vi "LEBITplc.PenningSetValue.vi"(0 "i ref in":refnum<vi>, 1 "Nickname in":string, 2 "i attribute in":T1, 3 "value":dbl, 4 "index in":i32, 5 "error in":errorcluster) -> (13 "In Range?":bool, 14 "i ref out":refnum<vi>, 15 "Nicknames out":string[](array[string]), 16 "Index out":i32[](array[numeric]), 17 "values":dbl[](array[numeric]), 18 "Log Out?":bool[](array[boolean]), 19 "error out":errorcluster)   [LabVIEW 2014, in "LEBITplc.lvlib"]
uses:
  LEBITplc.lvlib
  LEBITplc.i attribute.ctl
panel:
  in  "file path":path=path "\\\\Projects\\proj1/lebit/Data Exchange/data/IonGuideControl/Conversion/MassConversion.txt"
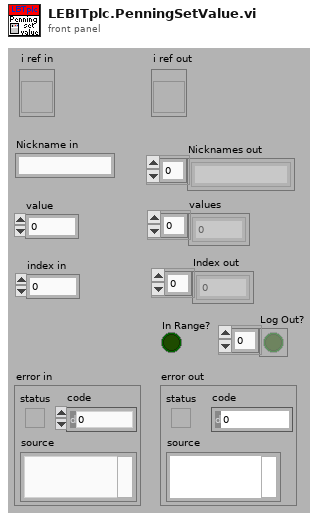
[diagram p1: front panel]
types:
  T1 = typedef "LEBITplc.lvlib/LEBITplc.i attribute.ctl" = cluster{"LLFLocation":string, "SetFileLocation":string, "nickNames":string[], "setValuePLCServiceID":i32[], "GUIServiceID":i32[], "monValuePLC":string[], "SetValueServiceID":i32[], "MonValueServiceID":i32[], "SetValue":dbl[][], "SetValueMin":dbl[], "SetValueMax":dbl[], "SetValueInfoServiceID":i32[], "GUINames":string[], "ListOfBases":string[], "Scale":dbl[], "Offset":dbl[], "setValuePLC":string[], "BaseName":string[], "ScaleServiceID":i32[], "OffsetServiceID":i32[], "AllPLCValues":string[], "CondSpecialArray":string[][], "CondSpecialIndex":i32[], "CondSpecialMonValue":dbl[], "RecentlyChanged":i32[], "SetFileLocationID":i32, "Dependent-Monitors":string[][], "LastLoadedFiles":string[], "IonGuideCalibLocation":string, "Monitor Dependent":string[], "Special":string[], "PLC?":bool[], "Start Date":string, "ListOfBasesServiceID":i32, "SETRA VISA resource":refnum<visa-resource-name>}
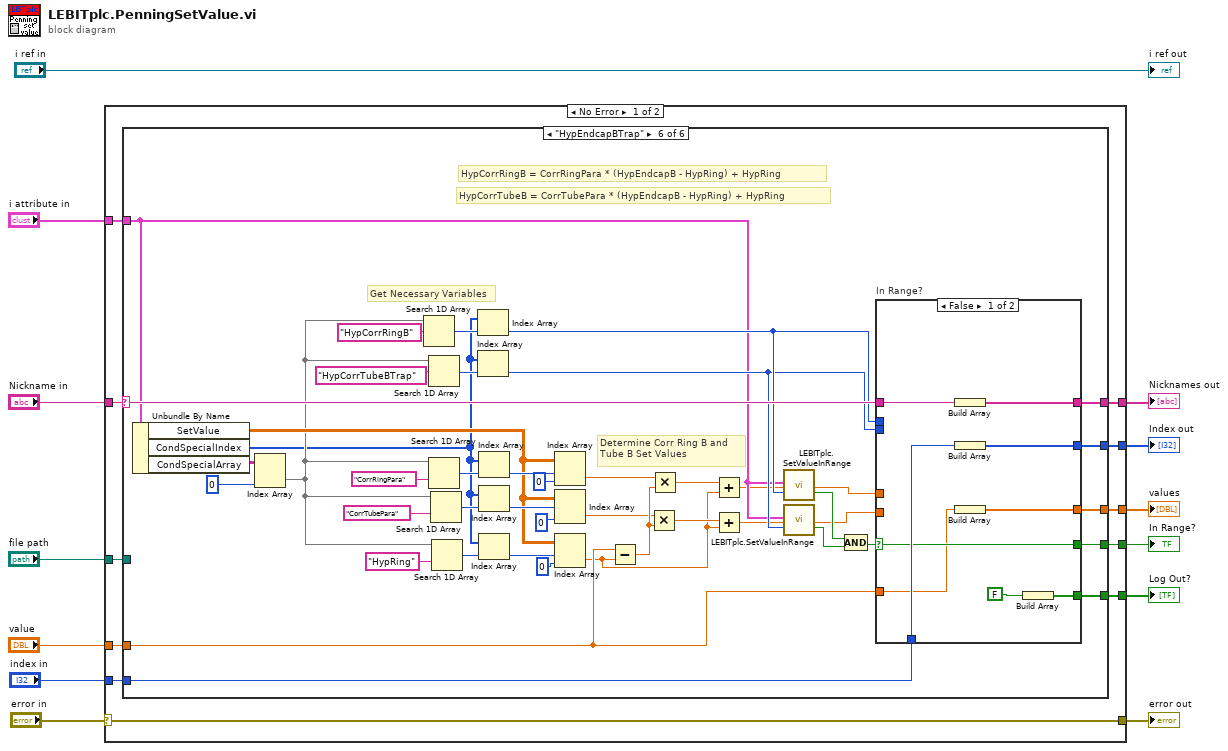
[diagram p0: block diagram]
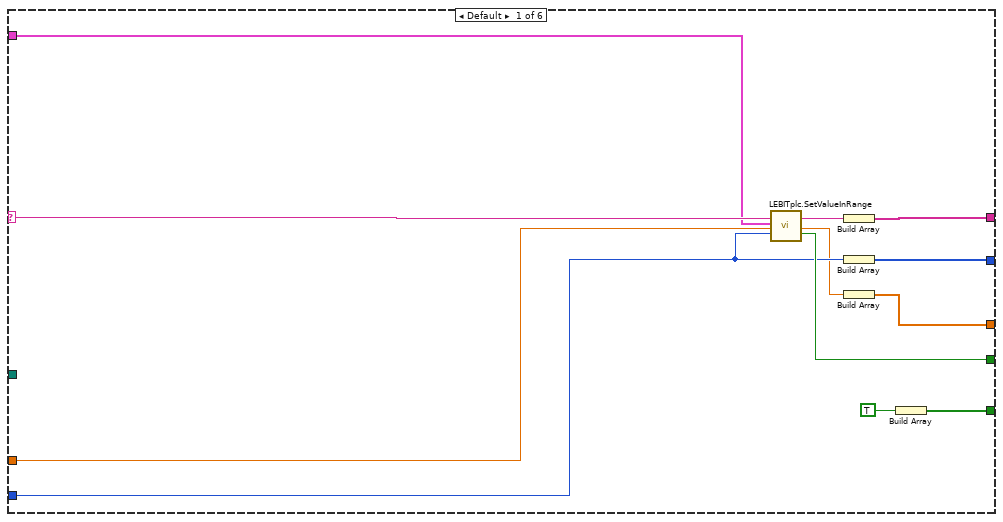
[diagram p2: hidden frame]
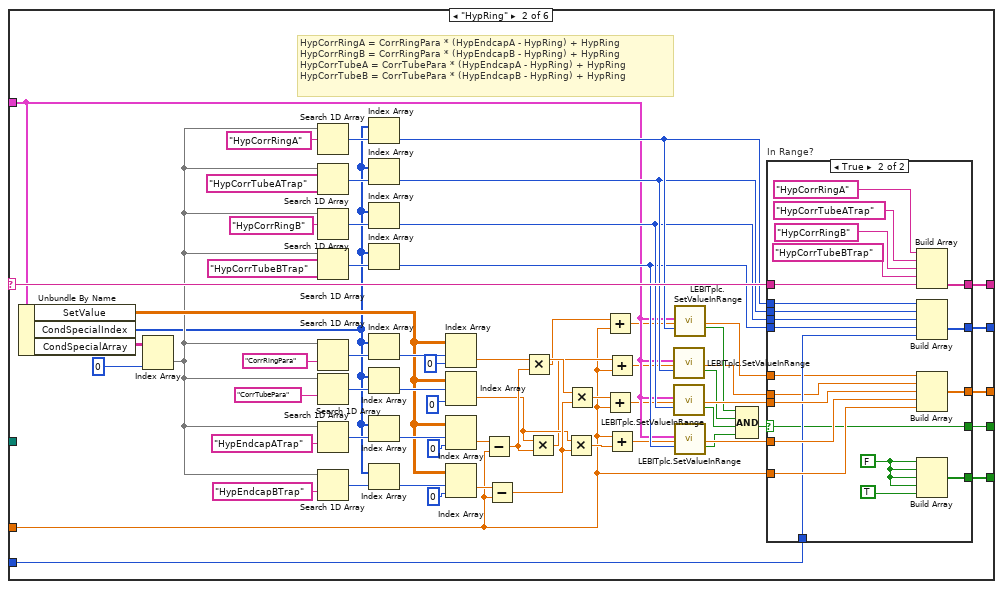
[diagram p3: hidden frame]
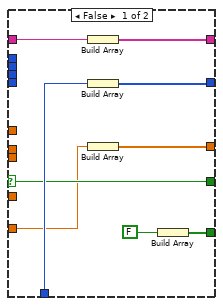
[diagram p4: hidden frame]
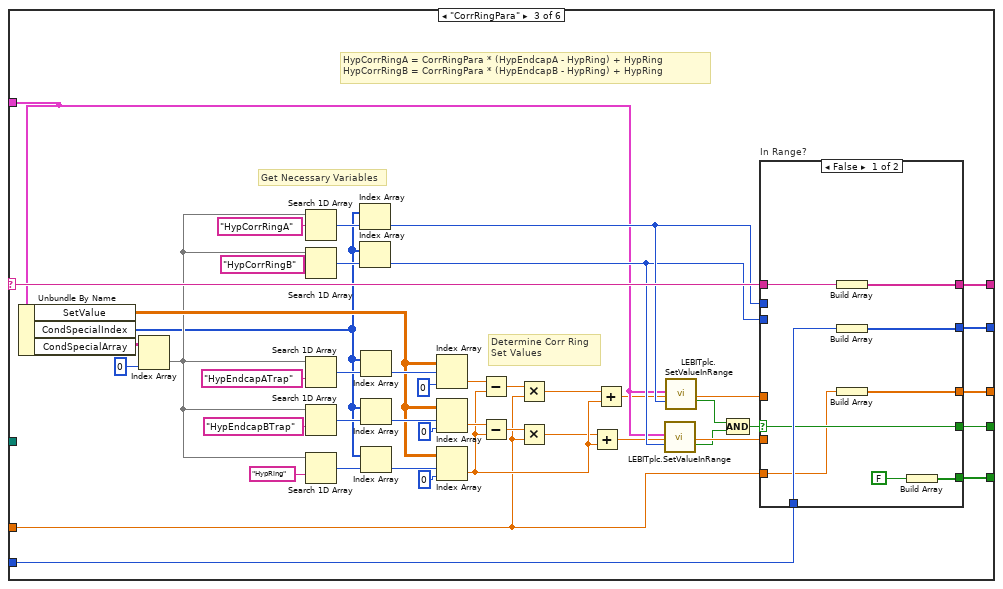
[diagram p5: hidden frame]
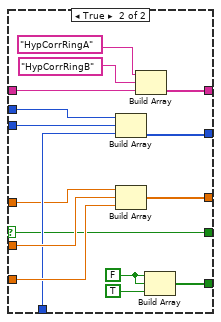
[diagram p6: hidden frame]
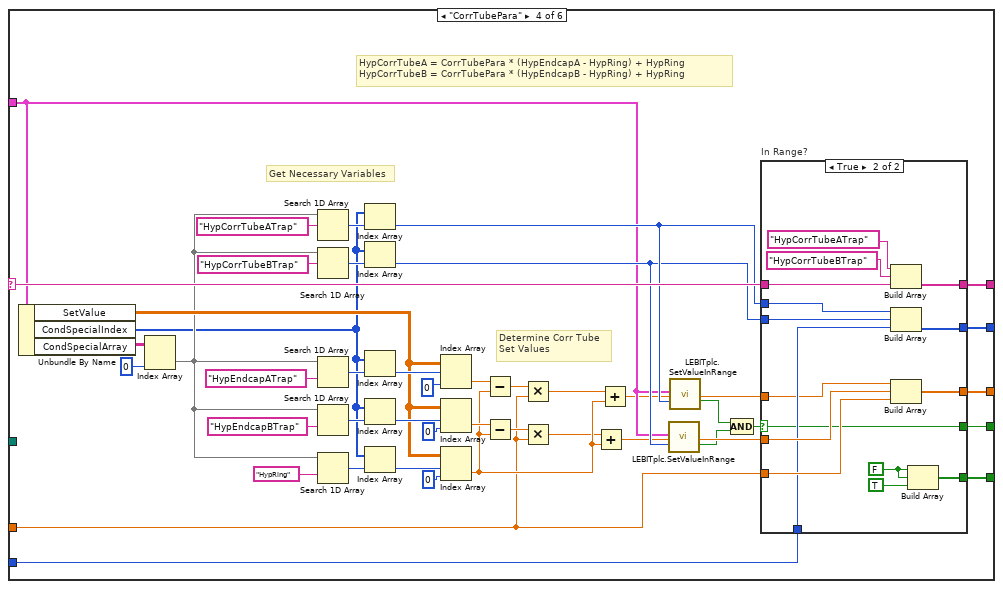
[diagram p7: hidden frame]
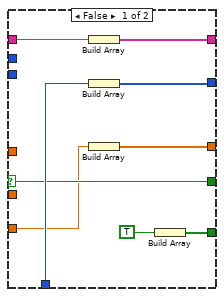
[diagram p8: hidden frame]
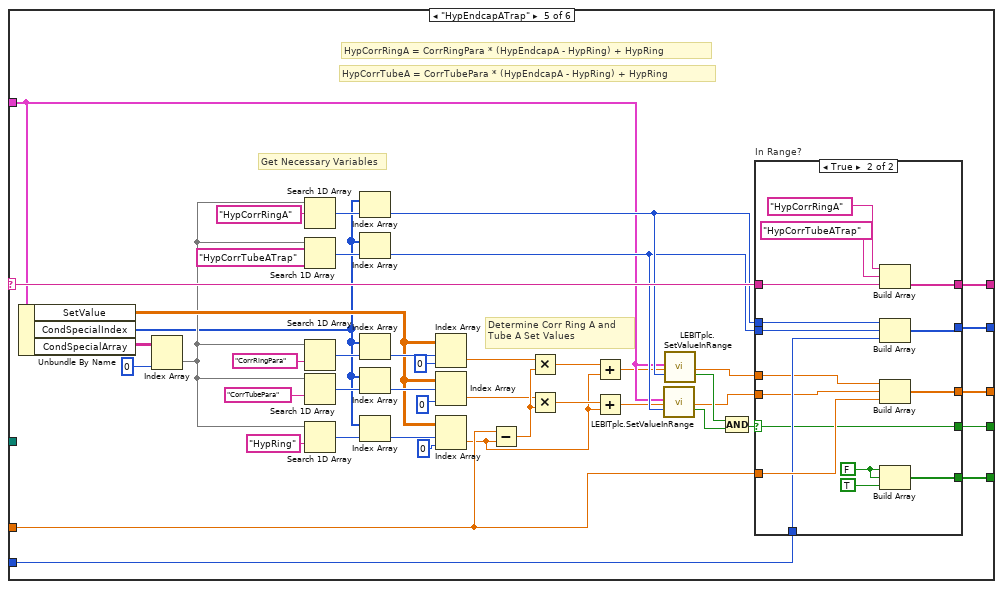
[diagram p9: hidden frame]
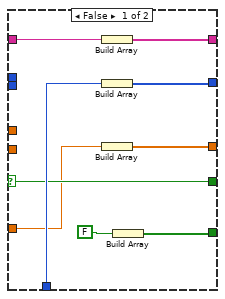
[diagram p10: hidden frame]
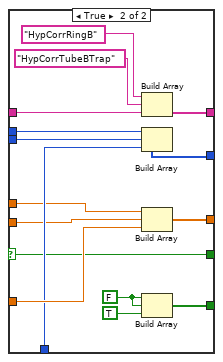
[diagram p11: hidden frame]
diagram:
  n1 = case shown="No Error" "error in" {
    selector: "error in" -> [w15 w415]
    tunnel: "Nickname in" -> [w24 _]
    tunnel: "i attribute in" -> [w23 _]
    tunnel: "value" -> [w22 _]
    tunnel: [w21 _] -> w10
    tunnel: [w20 _] -> w9
    tunnel: "file path" -> [w19 _]
    tunnel: "index in" -> [w18 _]
    tunnel: [w17 _] -> w6
    tunnel: [w16 _] -> w5
    tunnel: [w15 w415] -> w3
    tunnel: [w14 _] -> w1
    frame No Error {
      n2 = case shown="\"HypEndcapBTrap\"" w24 {
        selector: w24 -> [w32 w92 w172 w243 w312 w382]
        tunnel: w23 -> [w27 w50 w149 w220 w285 w355]
        tunnel: w22 -> [w30 w45 w134 w205 w277 w347]
        tunnel: [w36 w93 w173 w244 w313 w383] -> w21
        tunnel: [w35 w91 w171 w242 w311 w381] -> w20
        tunnel: w19 -> [_ _ _ _ _ _]
        tunnel: w18 -> [w31 w78 w162 w233 w302 w372]
        tunnel: [w34 w79 w163 w234 w303 w373] -> w17
        tunnel: [w33 w76 w160 w231 w300 w370] -> w16
        tunnel: [w25 w37 w133 w204 w275 w345] -> w14
        frame Default {
          n3 = call "LEBITplc.SetValueInRange.vi"("CommandName in"=w32, "i attribute in"=w27, "value in"=w30, "index of element"=w31) -> ("CommandName out"=w28:string, "value out"=w29:dbl, "In Range?"=w33:bool)  [unwired: 11 in, 2 out]
          n4 = Build Array(w28) -> (w35:string[])
          n5 = Build Array(w31) -> (w34:i32[])
          n6 = Build Array(w29) -> (w36:dbl[])
          n7 = Build Array(TRUE) -> (w25:bool[])
        }
        frame "HypRing" {
          # "HypCorrRingA = CorrRingPara * (HypEndcapA - HypRing) + HypRing\nHypCorrRingB = CorrRingPara * (HypEndcapB - HypRing) + HypRing\nHypCorrTubeA = CorrTubePara * (HypEndcapA - HypRing) + HypRing\nHypCorrTubeB = CorrTubePara * (HypEndcapB - HypRing) + HypRing"
          n8 = Unbundle By Name(w50) -> ("SetValue"=w71:dbl[][], "CondSpecialIndex"=w65:i32[], "CondSpecialArray"=w90:string[][])
          n9 = Index Array(array=w90, index (col)=0 ("index (row)")) -> (element=w66:string[])  [unwired: 1 in]
          n10 = Search 1D Array(1D array=w66, element="HypCorrRingA") -> (index of element=w68:i32)  [unwired: 1 in]
          n11 = Search 1D Array(1D array=w66, element="HypCorrTubeATrap") -> (index of element=w70:i32)  [unwired: 1 in]
          n12 = Search 1D Array(1D array=w66, element="HypCorrRingB") -> (index of element=w81:i32)  [unwired: 1 in]
          n13 = Search 1D Array(1D array=w66, element="HypCorrTubeBTrap") -> (index of element=w83:i32)  [unwired: 1 in]
          n14 = Search 1D Array(1D array=w66, element="CorrRingPara") -> (index of element=w89:i32)  [unwired: 1 in]
          n15 = Search 1D Array(1D array=w66, element="CorrTubePara") -> (index of element=w88:i32)  [unwired: 1 in]
          n16 = Search 1D Array(1D array=w66, element="HypEndcapATrap") -> (index of element=w87:i32)  [unwired: 1 in]
          n17 = Search 1D Array(1D array=w66, element="HypEndcapBTrap") -> (index of element=w73:i32)  [unwired: 1 in]
          n18 = Index Array(array=w65, index=w68) -> (element=w54:i32)
          n19 = Index Array(array=w65, index=w70) -> (element=w53:i32)
          n20 = Index Array(array=w65, index=w81) -> (element=w52:i32)
          n21 = Index Array(array=w65, index=w83) -> (element=w51:i32)
          n22 = Index Array(array=w65, index=w89) -> (element=w84:i32)
          n23 = Index Array(array=w65, index=w88) -> (element=w85:i32)
          n24 = Index Array(array=w65, index=w87) -> (element=w86:i32)
          n25 = Index Array(array=w65, index=w73) -> (element=w72:i32)
          n26 = Index Array(array=w71, index (row)=w84, index (col)=0 ("disabled index (col)")) -> (element=w62:dbl)
          n27 = Index Array(array=w71, index (row)=w85, index (col)=0 ("disabled index (col)")) -> (element=w59:dbl)
          n28 = Index Array(array=w71, index (row)=w86, index (col)=0 ("disabled index (col)")) -> (element=w63:dbl)
          n29 = Index Array(array=w71, index (row)=w72, index (col)=0 ("disabled index (col)")) -> (element=w64:dbl)
          n30 = Subtract(x=w63, y=w45) -> (x-y=w61:dbl)
          n31 = Subtract(x=w64, y=w45) -> (x-y=w60:dbl)
          n32 = Multiply(x=w62, y=w61) -> (x*y=w56:dbl)
          n33 = Multiply(x=w59, y=w61) -> (x*y=w55:dbl)
          n34 = Multiply(x=w59, y=w60) -> (x*y=w57:dbl)
          n35 = Multiply(x=w62, y=w60) -> (x*y=w58:dbl)
          n36 = Add(x=w56, y=w45) -> (x+y=w49:dbl)
          n37 = Add(x=w58, y=w45) -> (x+y=w47:dbl)
          n38 = Add(x=w55, y=w45) -> (x+y=w48:dbl)
          n39 = Add(x=w45, y=w57) -> (x+y=w46:dbl)
          n40 = call "LEBITplc.SetValueInRange.vi"("i attribute in"=w50, "value in"=w48, "index of element"=w53) -> ("value out"=w38:dbl, "In Range?"=w42:bool)  [unwired: 12 in, 3 out]
          n41 = call "LEBITplc.SetValueInRange.vi"("i attribute in"=w50, "value in"=w47, "index of element"=w52) -> ("value out"=w94:dbl, "In Range?"=w41:bool)  [unwired: 12 in, 3 out]
          n42 = call "LEBITplc.SetValueInRange.vi"("i attribute in"=w50, "value in"=w49, "index of element"=w54) -> ("value out"=w39:dbl, "In Range?"=w43:bool)  [unwired: 12 in, 3 out]
          n43 = call "LEBITplc.SetValueInRange.vi"("i attribute in"=w50, "value in"=w46, "index of element"=w51) -> ("value out"=w95:dbl, "In Range?"=w40:bool)  [unwired: 12 in, 3 out]
          n44 = Compound Arithmetic op=AND(w43, w42, w41, w40) -> (w44:bool)
          n45 = case "In Range?" shown="True" w44 {
            selector: w44 -> [w106 w124]
            tunnel: w45 -> [w105 w130]
            tunnel: w95 -> [_ w131]
            tunnel: w94 -> [_ w132]
            tunnel: [w104 w129] -> w93
            tunnel: w92 -> [w109 w128]
            tunnel: [w110 w127] -> w91
            tunnel: [w108 w126] -> w79
            tunnel: w78 -> [w107 w125]
            tunnel: [w106 w124] -> w76
            tunnel: w54 -> [_ w119]
            tunnel: w53 -> [_ w118]
            tunnel: w52 -> [_ w117]
            tunnel: w51 -> [_ w116]
            tunnel: w39 -> [_ w115]
            tunnel: w38 -> [_ w114]
            tunnel: [w102 w111] -> w37
            frame False {
              n46 = Build Array(w109) -> (w110:string[])
              n47 = Build Array(w107) -> (w108:i32[])
              n48 = Build Array(w105) -> (w104:dbl[])
              n49 = Build Array(FALSE) -> (w102:bool[])
            }
            frame True {
              w112 = FALSE
              n50 = Build Array("HypCorrRingA" ("element"), "HypCorrTubeATrap" ("element"), "HypCorrRingB" ("element"), "HypCorrTubeBTrap" ("element"), w128) -> (w127:string[])
              n51 = Build Array(w119, w118, w117, w116, w125) -> (w126:i32[])
              n52 = Build Array(w115, w114, w132, w131, w130) -> (w129:dbl[])
              n53 = Build Array(w112, w112, w112, w112, TRUE) -> (w111:bool[])
            }
          }
        }
        frame "CorrRingPara" {
          # "HypCorrRingA = CorrRingPara * (HypEndcapA - HypRing) + HypRing\nHypCorrRingB = CorrRingPara * (HypEndcapB - HypRing) + HypRing"
          # "Determine Corr Ring\nSet Values"
          # "Get Necessary Variables"
          n54 = Unbundle By Name(w149) -> ("SetValue"=w155:dbl[][], "CondSpecialIndex"=w142:i32[], "CondSpecialArray"=w170:string[][])
          n55 = Index Array(array=w170, index (col)=0 ("index (row)")) -> (element=w152:string[])  [unwired: 1 in]
          n56 = Search 1D Array(1D array=w152, element="HypCorrRingA") -> (index of element=w154:i32)  [unwired: 1 in]
          n57 = Search 1D Array(1D array=w152, element="HypCorrRingB") -> (index of element=w165:i32)  [unwired: 1 in]
          n58 = Search 1D Array(1D array=w152, element="HypEndcapATrap") -> (index of element=w169:i32)  [unwired: 1 in]
          n59 = Search 1D Array(1D array=w152, element="HypEndcapBTrap") -> (index of element=w168:i32)  [unwired: 1 in]
          n60 = Search 1D Array(1D array=w152, element="HypRing") -> (index of element=w157:i32)  [unwired: 1 in]
          n61 = Index Array(array=w142, index=w154) -> (element=w151:i32)
          n62 = Index Array(array=w142, index=w165) -> (element=w150:i32)
          n63 = Index Array(array=w142, index=w169) -> (element=w166:i32)
          n64 = Index Array(array=w142, index=w168) -> (element=w167:i32)
          n65 = Index Array(array=w142, index=w157) -> (element=w156:i32)
          n66 = Index Array(array=w155, index (row)=w166, index (col)=0 ("disabled index (col)")) -> (element=w141:dbl)
          n67 = Index Array(array=w155, index (row)=w167, index (col)=0 ("disabled index (col)")) -> (element=w140:dbl)
          n68 = Index Array(array=w155, index (row)=w156, index (col)=0 ("disabled index (col)")) -> (element=w139:dbl)
          n69 = Subtract(x=w141, y=w139) -> (x-y=w138:dbl)
          n70 = Subtract(x=w140, y=w139) -> (x-y=w137:dbl)
          n71 = Multiply(x=w138, y=w134) -> (x*y=w136:dbl)
          n72 = Multiply(x=w137, y=w134) -> (x*y=w135:dbl)
          n73 = Add(x=w135, y=w139) -> (x+y=w147:dbl)
          n74 = Add(x=w136, y=w139) -> (x+y=w148:dbl)
          n75 = call "LEBITplc.SetValueInRange.vi"("i attribute in"=w149, "value in"=w147, "index of element"=w150) -> ("value out"=w174:dbl, "In Range?"=w144:bool)  [unwired: 12 in, 3 out]
          n76 = call "LEBITplc.SetValueInRange.vi"("i attribute in"=w149, "value in"=w148, "index of element"=w151) -> ("value out"=w143:dbl, "In Range?"=w145:bool)  [unwired: 12 in, 3 out]
          n77 = Compound Arithmetic op=AND(w145, w144) -> (w146:bool)
          n78 = case "In Range?" shown="False" w146 {
            selector: w146 -> [w183 w196]
            tunnel: w134 -> [w182 w202]
            tunnel: w174 -> [_ w203]
            tunnel: [w181 w201] -> w173
            tunnel: w172 -> [w186 w200]
            tunnel: [w187 w199] -> w171
            tunnel: [w185 w198] -> w163
            tunnel: w162 -> [w184 w197]
            tunnel: [w183 w196] -> w160
            tunnel: w151 -> [_ w193]
            tunnel: w150 -> [_ w192]
            tunnel: w143 -> [_ w191]
            tunnel: [w179 w188] -> w133
            frame False {
              n79 = Build Array(w186) -> (w187:string[])
              n80 = Build Array(w184) -> (w185:i32[])
              n81 = Build Array(w182) -> (w181:dbl[])
              n82 = Build Array(FALSE) -> (w179:bool[])
            }
            frame True {
              w189 = FALSE
              n83 = Build Array(w193, w192, w197) -> (w198:i32[])
              n84 = Build Array(w191, w203, w202) -> (w201:dbl[])
              n85 = Build Array("HypCorrRingA" ("element"), "HypCorrRingB" ("element"), w200) -> (w199:string[])
              n86 = Build Array(w189, w189, TRUE) -> (w188:bool[])
            }
          }
        }
        frame "CorrTubePara" {
          # "HypCorrTubeA = CorrTubePara * (HypEndcapA - HypRing) + HypRing\nHypCorrTubeB = CorrTubePara * (HypEndcapB - HypRing) + HypRing"
          # "Determine Corr Tube\nSet Values"
          # "Get Necessary Variables"
          n87 = Unbundle By Name(w220) -> ("SetValue"=w226:dbl[][], "CondSpecialIndex"=w213:i32[], "CondSpecialArray"=w241:string[][])
          n88 = Index Array(array=w241, index (col)=0 ("index (row)")) -> (element=w223:string[])  [unwired: 1 in]
          n89 = Search 1D Array(1D array=w223, element="HypCorrTubeATrap") -> (index of element=w225:i32)  [unwired: 1 in]
          n90 = Search 1D Array(1D array=w223, element="HypCorrTubeBTrap") -> (index of element=w236:i32)  [unwired: 1 in]
          n91 = Search 1D Array(1D array=w223, element="HypEndcapATrap") -> (index of element=w240:i32)  [unwired: 1 in]
          n92 = Search 1D Array(1D array=w223, element="HypEndcapBTrap") -> (index of element=w239:i32)  [unwired: 1 in]
          n93 = Search 1D Array(1D array=w223, element="HypRing") -> (index of element=w228:i32)  [unwired: 1 in]
          n94 = Index Array(array=w213, index=w225) -> (element=w222:i32)
          n95 = Index Array(array=w213, index=w236) -> (element=w221:i32)
          n96 = Index Array(array=w213, index=w240) -> (element=w237:i32)
          n97 = Index Array(array=w213, index=w239) -> (element=w238:i32)
          n98 = Index Array(array=w213, index=w228) -> (element=w227:i32)
          n99 = Index Array(array=w226, index (row)=w237, index (col)=0 ("disabled index (col)")) -> (element=w212:dbl)
          n100 = Index Array(array=w226, index (row)=w238, index (col)=0 ("disabled index (col)")) -> (element=w211:dbl)
          n101 = Index Array(array=w226, index (row)=w227, index (col)=0 ("disabled index (col)")) -> (element=w210:dbl)
          n102 = Subtract(x=w212, y=w210) -> (x-y=w209:dbl)
          n103 = Subtract(x=w211, y=w210) -> (x-y=w208:dbl)
          n104 = Multiply(x=w209, y=w205) -> (x*y=w207:dbl)
          n105 = Multiply(x=w208, y=w205) -> (x*y=w206:dbl)
          n106 = Add(x=w206, y=w210) -> (x+y=w218:dbl)
          n107 = Add(x=w207, y=w210) -> (x+y=w219:dbl)
          n108 = call "LEBITplc.SetValueInRange.vi"("i attribute in"=w220, "value in"=w218, "index of element"=w221) -> ("value out"=w245:dbl, "In Range?"=w215:bool)  [unwired: 12 in, 3 out]
          n109 = call "LEBITplc.SetValueInRange.vi"("i attribute in"=w220, "value in"=w219, "index of element"=w222) -> ("value out"=w214:dbl, "In Range?"=w216:bool)  [unwired: 12 in, 3 out]
          n110 = Compound Arithmetic op=AND(w216, w215) -> (w217:bool)
          n111 = case "In Range?" shown="True" w217 {
            selector: w217 -> [w254 w267]
            tunnel: w205 -> [w253 w273]
            tunnel: w245 -> [_ w274]
            tunnel: [w252 w272] -> w244
            tunnel: w243 -> [w257 w271]
            tunnel: [w258 w270] -> w242
            tunnel: [w256 w269] -> w234
            tunnel: w233 -> [w255 w268]
            tunnel: [w254 w267] -> w231
            tunnel: w222 -> [_ w264]
            tunnel: w221 -> [_ w263]
            tunnel: w214 -> [_ w262]
            tunnel: [w250 w259] -> w204
            frame False {
              n112 = Build Array(w257) -> (w258:string[])
              n113 = Build Array(w255) -> (w256:i32[])
              n114 = Build Array(w253) -> (w252:dbl[])
              n115 = Build Array(TRUE) -> (w250:bool[])
            }
            frame True {
              w260 = FALSE
              n116 = Build Array("HypCorrTubeATrap" ("element"), "HypCorrTubeBTrap" ("element"), w271) -> (w270:string[])
              n117 = Build Array(w264, w263, w268) -> (w269:i32[])
              n118 = Build Array(w262, w274, w273) -> (w272:dbl[])
              n119 = Build Array(w260, w260, TRUE) -> (w259:bool[])
            }
          }
        }
        frame "HypEndcapATrap" {
          # "HypCorrTubeA = CorrTubePara * (HypEndcapA - HypRing) + HypRing"
          # "HypCorrRingA = CorrRingPara * (HypEndcapA - HypRing) + HypRing"
          # "Determine Corr Ring A and \nTube A Set Values"
          # "Get Necessary Variables"
          n120 = Unbundle By Name(w285) -> ("SetValue"=w299:dbl[][], "CondSpecialIndex"=w293:i32[], "CondSpecialArray"=w310:string[][])
          n121 = Index Array(array=w310, index (col)=0 ("index (row)")) -> (element=w294:string[])  [unwired: 1 in]
          n122 = Search 1D Array(1D array=w294, element="HypCorrRingA") -> (index of element=w296:i32)  [unwired: 1 in]
          n123 = Search 1D Array(1D array=w294, element="HypCorrTubeATrap") -> (index of element=w298:i32)  [unwired: 1 in]
          n124 = Search 1D Array(1D array=w294, element="CorrRingPara") -> (index of element=w309:i32)  [unwired: 1 in]
          n125 = Search 1D Array(1D array=w294, element="CorrTubePara") -> (index of element=w308:i32)  [unwired: 1 in]
          n126 = Search 1D Array(1D array=w294, element="HypRing") -> (index of element=w307:i32)  [unwired: 1 in]
          n127 = Index Array(array=w293, index=w296) -> (element=w287:i32)
          n128 = Index Array(array=w293, index=w298) -> (element=w286:i32)
          n129 = Index Array(array=w293, index=w309) -> (element=w304:i32)
          n130 = Index Array(array=w293, index=w308) -> (element=w305:i32)
          n131 = Index Array(array=w293, index=w307) -> (element=w306:i32)
          n132 = Index Array(array=w299, index (row)=w304, index (col)=0 ("disabled index (col)")) -> (element=w292:dbl)
          n133 = Index Array(array=w299, index (row)=w305, index (col)=0 ("disabled index (col)")) -> (element=w290:dbl)
          n134 = Index Array(array=w299, index (row)=w306, index (col)=0 ("disabled index (col)")) -> (element=w276:dbl)
          n135 = Subtract(x=w277, y=w276) -> (x-y=w291:dbl)
          n136 = Multiply(x=w292, y=w291) -> (x*y=w289:dbl)
          n137 = Multiply(x=w290, y=w291) -> (x*y=w288:dbl)
          n138 = Add(x=w289, y=w276) -> (x+y=w284:dbl)
          n139 = Add(x=w288, y=w276) -> (x+y=w283:dbl)
          n140 = call "LEBITplc.SetValueInRange.vi"("i attribute in"=w285, "value in"=w283, "index of element"=w286) -> ("value out"=w278:dbl, "In Range?"=w280:bool)  [unwired: 12 in, 3 out]
          n141 = call "LEBITplc.SetValueInRange.vi"("i attribute in"=w285, "value in"=w284, "index of element"=w287) -> ("value out"=w279:dbl, "In Range?"=w281:bool)  [unwired: 12 in, 3 out]
          n142 = Compound Arithmetic op=AND(w281, w280) -> (w282:bool)
          n143 = case "In Range?" shown="True" w282 {
            selector: w282 -> [w324 w338]
            tunnel: w277 -> [w323 w344]
            tunnel: [w322 w343] -> w313
            tunnel: w312 -> [w327 w342]
            tunnel: [w328 w341] -> w311
            tunnel: [w326 w340] -> w303
            tunnel: w302 -> [w325 w339]
            tunnel: [w324 w338] -> w300
            tunnel: w287 -> [_ w335]
            tunnel: w286 -> [_ w334]
            tunnel: w279 -> [_ w333]
            tunnel: w278 -> [_ w332]
            tunnel: [w321 w329] -> w275
            frame False {
              n144 = Build Array(w327) -> (w328:string[])
              n145 = Build Array(w325) -> (w326:i32[])
              n146 = Build Array(w323) -> (w322:dbl[])
              n147 = Build Array(FALSE) -> (w321:bool[])
            }
            frame True {
              w330 = FALSE
              n148 = Build Array("HypCorrRingA" ("element"), "HypCorrTubeATrap" ("element"), w342) -> (w341:string[])
              n149 = Build Array(w335, w334, w339) -> (w340:i32[])
              n150 = Build Array(w333, w332, w344) -> (w343:dbl[])
              n151 = Build Array(w330, w330, TRUE) -> (w329:bool[])
            }
          }
        }
        frame "HypEndcapBTrap" {
          # "HypCorrTubeB = CorrTubePara * (HypEndcapB - HypRing) + HypRing"
          # "HypCorrRingB = CorrRingPara * (HypEndcapB - HypRing) + HypRing"
          # "Determine Corr Ring B and \nTube B Set Values"
          # "Get Necessary Variables"
          n152 = Unbundle By Name(w355) -> ("SetValue"=w369:dbl[][], "CondSpecialIndex"=w363:i32[], "CondSpecialArray"=w380:string[][])
          n153 = Index Array(array=w380, index (col)=0 ("index (row)")) -> (element=w364:string[])  [unwired: 1 in]
          n154 = Search 1D Array(1D array=w364, element="HypCorrRingB") -> (index of element=w366:i32)  [unwired: 1 in]
          n155 = Search 1D Array(1D array=w364, element="HypCorrTubeBTrap") -> (index of element=w368:i32)  [unwired: 1 in]
          n156 = Search 1D Array(1D array=w364, element="CorrRingPara") -> (index of element=w379:i32)  [unwired: 1 in]
          n157 = Search 1D Array(1D array=w364, element="CorrTubePara") -> (index of element=w378:i32)  [unwired: 1 in]
          n158 = Search 1D Array(1D array=w364, element="HypRing") -> (index of element=w377:i32)  [unwired: 1 in]
          n159 = Index Array(array=w363, index=w366) -> (element=w357:i32)
          n160 = Index Array(array=w363, index=w368) -> (element=w356:i32)
          n161 = Index Array(array=w363, index=w379) -> (element=w374:i32)
          n162 = Index Array(array=w363, index=w378) -> (element=w375:i32)
          n163 = Index Array(array=w363, index=w377) -> (element=w376:i32)
          n164 = Index Array(array=w369, index (row)=w374, index (col)=0 ("disabled index (col)")) -> (element=w362:dbl)
          n165 = Index Array(array=w369, index (row)=w375, index (col)=0 ("disabled index (col)")) -> (element=w360:dbl)
          n166 = Index Array(array=w369, index (row)=w376, index (col)=0 ("disabled index (col)")) -> (element=w346:dbl)
          n167 = Subtract(x=w347, y=w346) -> (x-y=w361:dbl)
          n168 = Multiply(x=w360, y=w361) -> (x*y=w358:dbl)
          n169 = Multiply(x=w362, y=w361) -> (x*y=w359:dbl)
          n170 = Add(x=w359, y=w346) -> (x+y=w354:dbl)
          n171 = Add(x=w358, y=w346) -> (x+y=w353:dbl)
          n172 = call "LEBITplc.SetValueInRange.vi"("i attribute in"=w355, "value in"=w354, "index of element"=w357) -> ("value out"=w349:dbl, "In Range?"=w351:bool)  [unwired: 12 in, 3 out]
          n173 = call "LEBITplc.SetValueInRange.vi"("i attribute in"=w355, "value in"=w353, "index of element"=w356) -> ("value out"=w348:dbl, "In Range?"=w350:bool)  [unwired: 12 in, 3 out]
          n174 = Compound Arithmetic op=AND(w351, w350) -> (w352:bool)
          n175 = case "In Range?" shown="False" w352 {
            selector: w352 -> [w394 w408]
            tunnel: w347 -> [w393 w414]
            tunnel: [w392 w413] -> w383
            tunnel: w382 -> [w397 w412]
            tunnel: [w398 w411] -> w381
            tunnel: [w396 w410] -> w373
            tunnel: w372 -> [w395 w409]
            tunnel: [w394 w408] -> w370
            tunnel: w357 -> [_ w405]
            tunnel: w356 -> [_ w404]
            tunnel: w349 -> [_ w403]
            tunnel: w348 -> [_ w402]
            tunnel: [w390 w399] -> w345
            frame False {
              n176 = Build Array(w397) -> (w398:string[])
              n177 = Build Array(w395) -> (w396:i32[])
              n178 = Build Array(w393) -> (w392:dbl[])
              n179 = Build Array(FALSE) -> (w390:bool[])
            }
            frame True {
              w400 = FALSE
              n180 = Build Array("HypCorrRingB" ("element"), "HypCorrTubeBTrap" ("element"), w412) -> (w411:string[])
              n181 = Build Array(w405, w404, w409) -> (w410:i32[])
              n182 = Build Array(w403, w402, w414) -> (w413:dbl[])
              n183 = Build Array(w400, w400, TRUE) -> (w399:bool[])
            }
          }
        }
      }
    }
    frame Error {
    }
  }
  "values" <- w10
  "Nicknames out" <- w9
  "Index out" <- w6
  "In Range?" <- w5
  "error out" <- w3
  "Log Out?" <- w1
  "i ref out" <- "i ref in"
